vi "Configure Limits.vi"(0 "VISA resource name":refnum<visa-resource-name>, 1 "Limit Number (Limit 1)":u16(ring) items=["Limit 1", "Limit 2"], 2 "Enable Selected Limit (F: Disable)":bool, 3 "Upper Limit (1)":dbl=1.0, 4 "Lower Limit (-1)":dbl=-1.0, 5 "error in (no error)":errorcluster, 6 "Channel List (Empty)":string, 7 "Enable Limit Auto-Clear (True)":bool=TRUE) -> (14 "VISA resource name out":refnum<visa-resource-name>, 19 "error out":errorcluster)   [LabVIEW 2020, in "Keithley 27XX.lvlib"]
doc: "This VI allows you to set the high and low bounds for limit 1 and limit 2."
uses:
  Keithley 27XX.lvlib
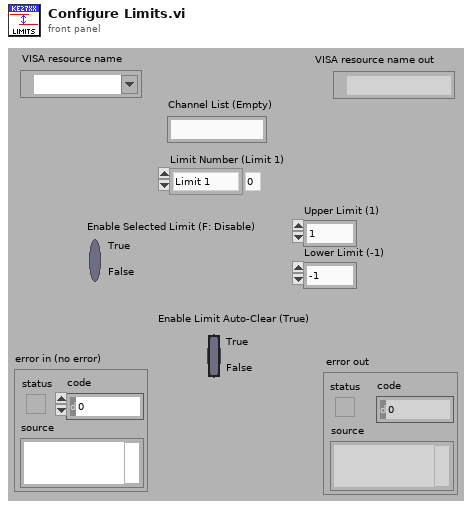
[diagram p1: front panel]
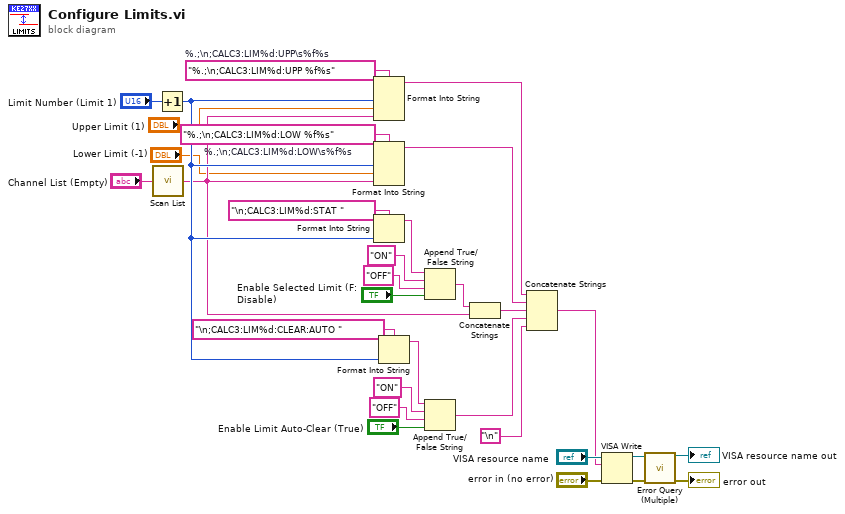
[diagram p0: block diagram]
diagram:
  w25 = "%.;\n;CALC3:LIM%d:LOW %f%s"  # %.;\n;CALC3:LIM%d:LOW\s%f%s
  w30 = "%.;\n;CALC3:LIM%d:UPP %f%s"  # %.;\n;CALC3:LIM%d:UPP\s%f%s
  n1 = call "Scan List.vi"("Scan List (Empty)"="Channel List (Empty)") -> ("Scan List Out"=w24:string)  [unwired: 14 in]
  n2 = Increment(x="Limit Number (Limit 1)") -> (x+1=w28:u16)
  n3 = Format Into String(format string=w30, w28, "Upper Limit (1)", w24) -> (resulting string=w12:string)  [unwired: 2 in, 1 out]
  n4 = Format Into String(format string=w25, w28, "Lower Limit (-1)", w24) -> (resulting string=w11:string)  [unwired: 2 in, 1 out]
  n5 = Format Into String(format string="\n;CALC3:LIM%d:STAT ", w28) -> (resulting string=w18:string)  [unwired: 2 in, 1 out]
  n6 = Format Into String(format string="\n;CALC3:LIM%d:CLEAR:AUTO ", w28) -> (resulting string=w13:string)  [unwired: 2 in, 1 out]
  n7 = Append True/False String(1:"Enable Selected Limit (F: Disable)", 2:"OFF", 3:"ON", 4:w18) -> (0:w17:string)
  n8 = Append True/False String(1:"Enable Limit Auto-Clear (True)", 2:"OFF", 3:"ON", 4:w13) -> (0:w9:string)
  n9 = Concatenate Strings(w17, w24) -> (w10:string)
  n10 = Concatenate Strings(w12, w11, w10, w9, "\n") -> (w6:string)
  n11 = VISA Write(VISA resource name="VISA resource name", write buffer=w6, error in (no error)="error in (no error)") -> (VISA resource name out=w5:refnum<visa-resource-name>, error out=w4:errorcluster)  [unwired: 1 out]
  n12 = call "Error Query (Multiple).vi"("VISA resource name"=w5, "error in (no error)"=w4) -> ("VISA resource name out"=→"VISA resource name out":refnum<visa-resource-name>, "error out"=→"error out":errorcluster)  [unwired: 10 in, 2 out]
